vi "Test ZLG_CAN API.vi"() -> ()   [LabVIEW 2020]
doc: "ZLG_CAN API Tester."
uses:
  ZLG_CAN.lvlib
  <userlib>/_OpenG.lib/array/array.llb/Reverse 2D Array (String)__ogtk.vi
  CAN_CYCLE.vi
  Sources/Global_Variable/Global.vi
panel:
  in  "Test":bool
  in  "Recive_Wait":bool
  out "Cycle_VI":refnum<vi>[](array[refnum])
  in  "CAN_CYCLE":T1(array[cluster]) {"周期(ms)" min=1 format="%d ms"; "ID" format="0x%x"}
  in  "CAN_Recive_Data":string[][](table)
  in  "帧格式":enum8{"数据帧", "远程帧"}(ring)
  in  "帧类型":enum8{"标准帧", "扩展帧"}(ring)
  in  "SENT CAN":bool
  in  "CAN_Frame":string
  in  "ID":u32
  in  "SENT CAN CYCLE":bool
  out "CAN Opening？":bool
  in  "波特率":u32(ring)=11 items=["5Kbps", "10Kbps", "20Kbps", "40Kbps", "50Kbps", "80Kbps", "100Kbps", "125Kbps", "200Kbps", "250Kbps", "400Kbps", "500Kbps", "666Kbps", "800Kbps", "1000Kbps"]
  in  "Close_CAN":bool
  in  "Open_CAN":bool
  in  "通道":u32(ring) items=["0", "1"]
  in  "索引":u32(ring) items=["0", "1", "2", "3", "4", "5", "6", "7", "8"]
  in  "设备类型":u32(ring)=27 items=["PCI5121"=1, "PCI9810"=2, "USBCAN1"=3, "USBCAN2"=4, "PCI9820"=5, "PCI5110"=7, "PC104CAN"=11, "CANETUDP"=12, "PCI9840B"=14, "PC104C2"=15, "PCI9820I"=16, "CANETTCP"=17, "PCIE9221"=24, "PCI5010U"=19, "USBCAN_E_U"=20, "USBCAN_2E_U"=21, "PCI5020U"=22, "PCIE9120I"=27, "PCIE9110I"=28, "PCIE9140I"=29]
  in  "Show Block Diagram":bool
  in  "Stop Module":bool
  in  "Start Module":bool
  in  "Hide Module Panel":bool
  in  "Show Module Panel":bool
  out "Status":string
  out "Module Running?":bool
  # "This VI tests the API for the Module."
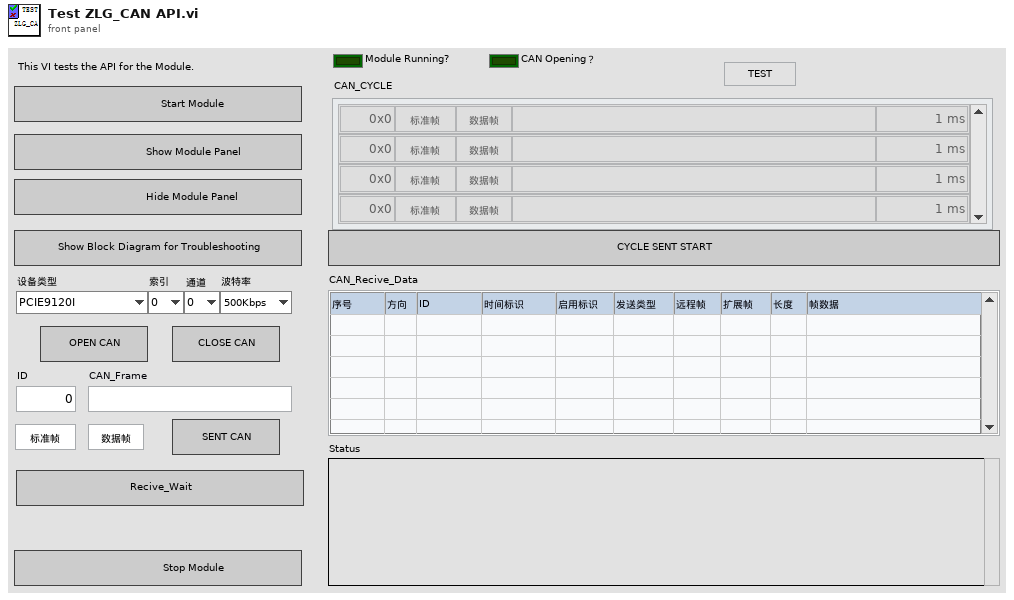
[diagram p1: front panel]
types:
  T1 = cluster{"ID":u32, "帧类型":enum8{"标准帧", "扩展帧"}, "帧格式":enum16{"数据帧", "远程帧"}, "帧数据":string, "周期(ms)":u32}[]
  T2 = typedef "ZLG_CAN.lvlib/Broadcast Events--cluster.ctl" = cluster{"Module Did Init":refnum<user-event>, "Status Updated":refnum<user-event>, "Error Reported":refnum<user-event>, "Module Did Stop":refnum<user-event>, "Update Module Execution Status":refnum<user-event>, "CAN_Recive":refnum<user-event>}
  T3 = enum32{"Invalid", "Standard", "Closed", "Hidden", "Minimized", "Maximized"}
  T4 = typedef "ZLG_CAN.lvlib/Start_CAN (Reply Payload)--cluster.ctl" = cluster{"Success":bool, "Start_CAN_error":errorcluster}
  T5 = typedef "ZLG_CAN.lvlib/CAN_Frame.ctl" = cluster{"[0]":u8, "[1]":u8, "[2]":u8, "[3]":u8, "[4]":u8, "[5]":u8, "[6]":u8, "[7]":u8}
  T6 = typedef "ZLG_CAN.lvlib/CAN_OBJ_R.ctl" = cluster{"ID":u32, "TimeStamp":u32, "TimeFlag":u8, "SendType":u8, "RemoteFlag":u8, "ExternFlag":u8, "DataLen":u8, "数值":u8, "数值":u8, "数值":u8, "数值":u8, "数值":u8, "数值":u8, "数值":u8, "数值":u8, "数值":u8, "数值":u8, "数值":u8}
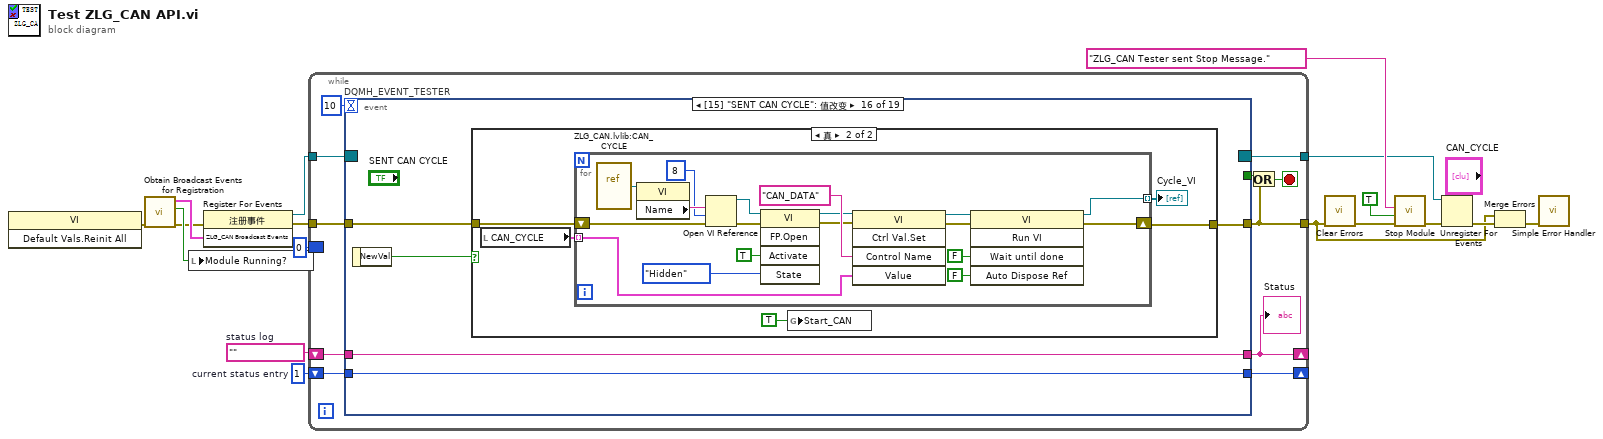
[diagram p0: block diagram]
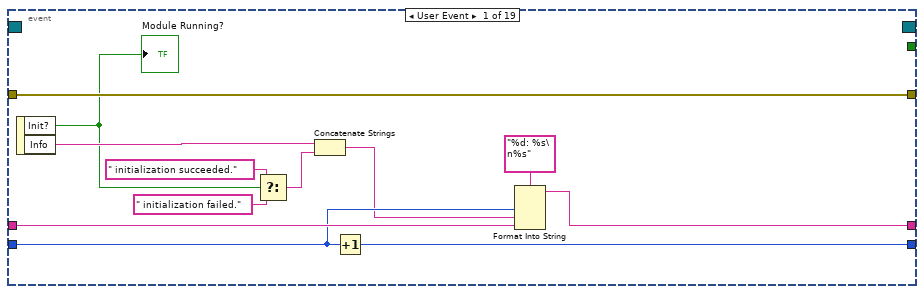
[diagram p2: hidden frame]
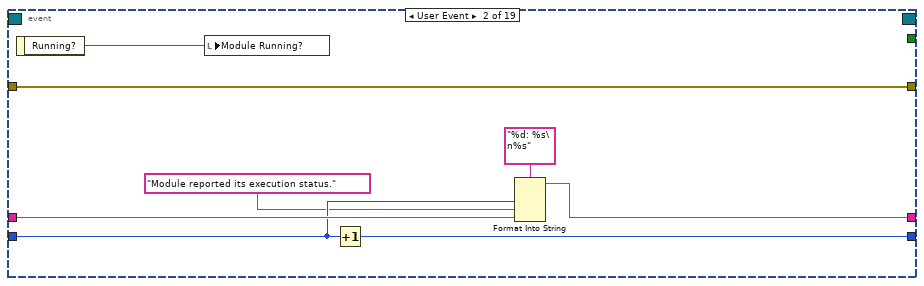
[diagram p3: hidden frame]
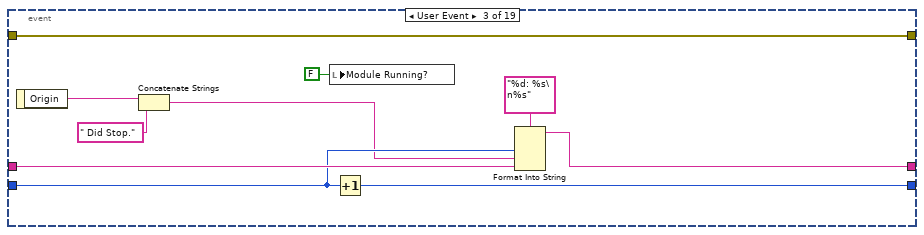
[diagram p4: hidden frame]
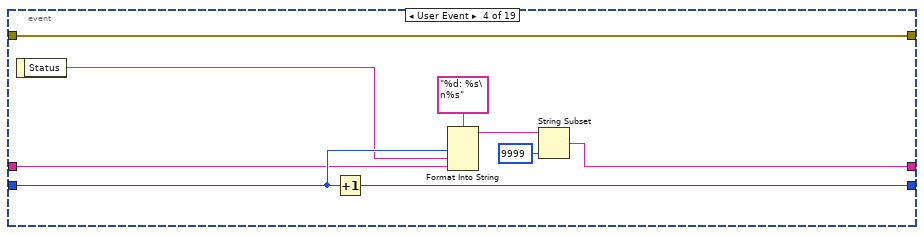
[diagram p5: hidden frame]
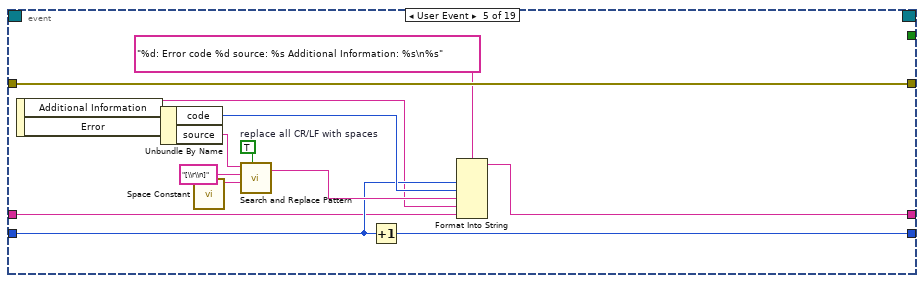
[diagram p6: hidden frame]
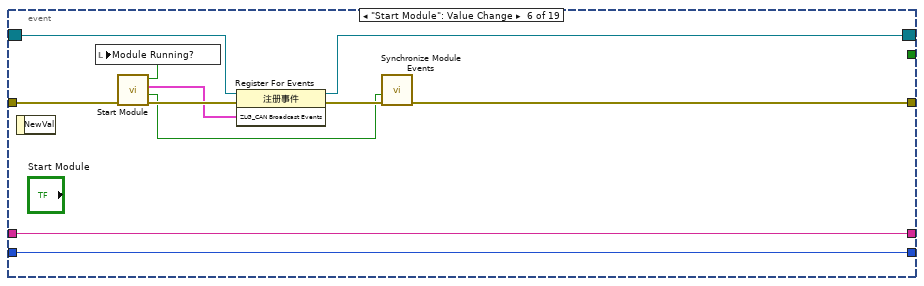
[diagram p7: hidden frame]
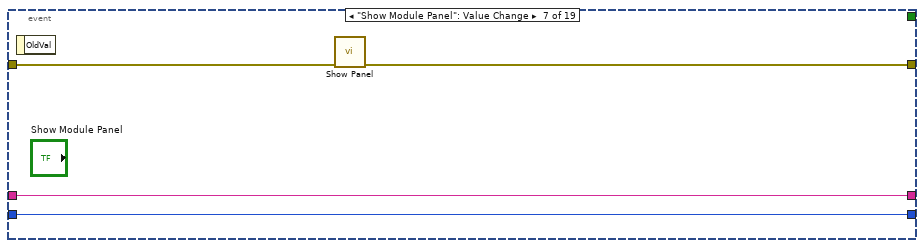
[diagram p8: hidden frame]
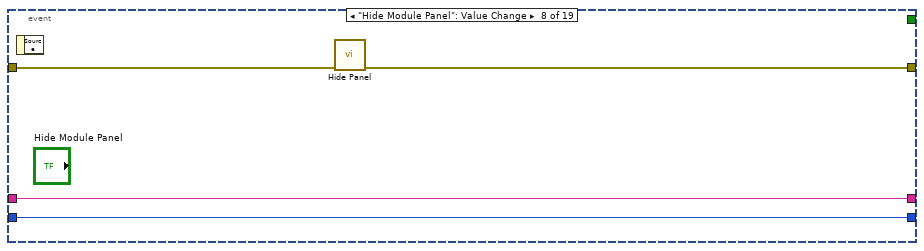
[diagram p9: hidden frame]
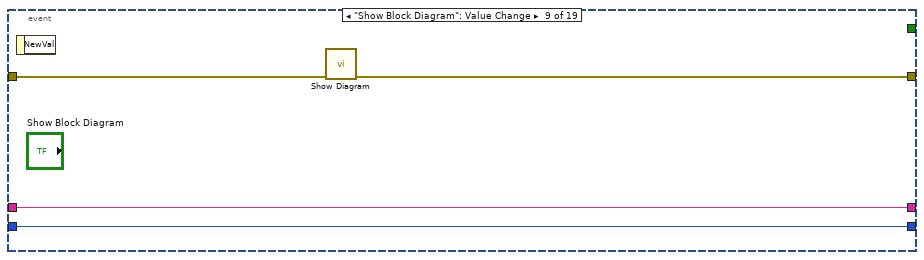
[diagram p10: hidden frame]
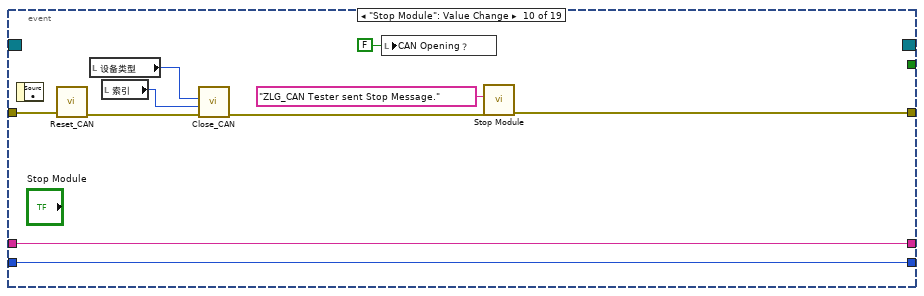
[diagram p11: hidden frame]
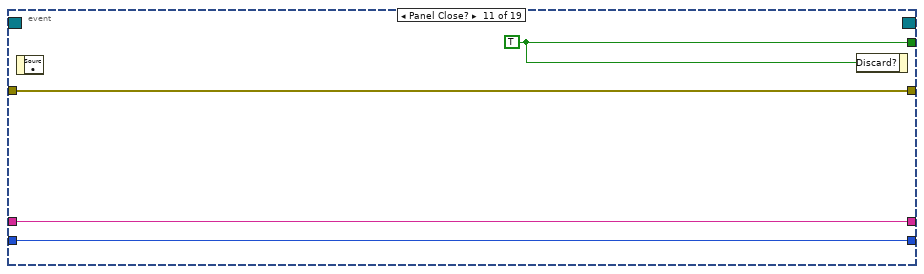
[diagram p12: hidden frame]
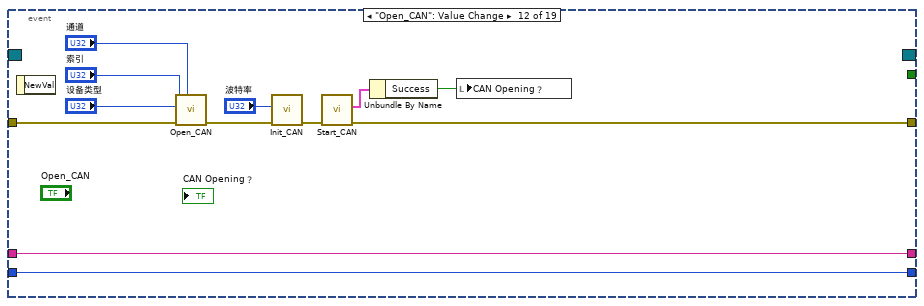
[diagram p13: hidden frame]
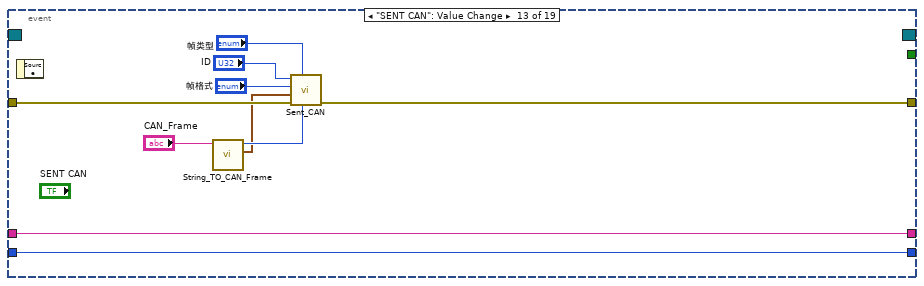
[diagram p14: hidden frame]
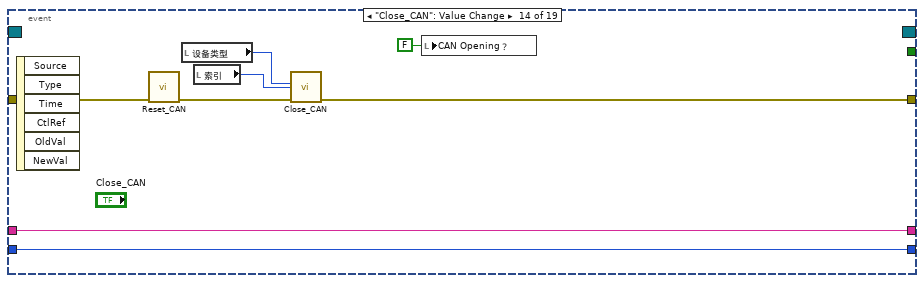
[diagram p15: hidden frame]
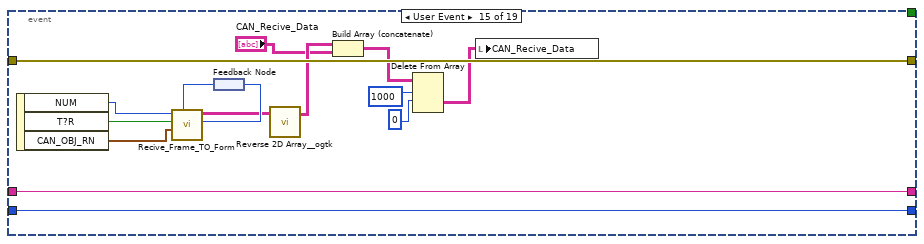
[diagram p16: hidden frame]
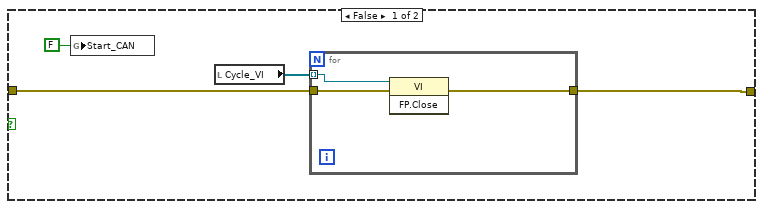
[diagram p17: hidden frame]
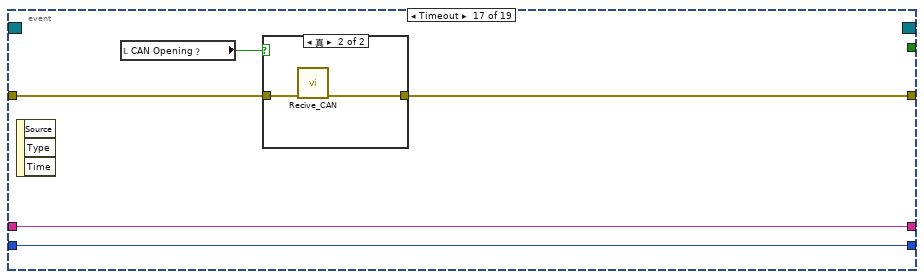
[diagram p18: hidden frame]
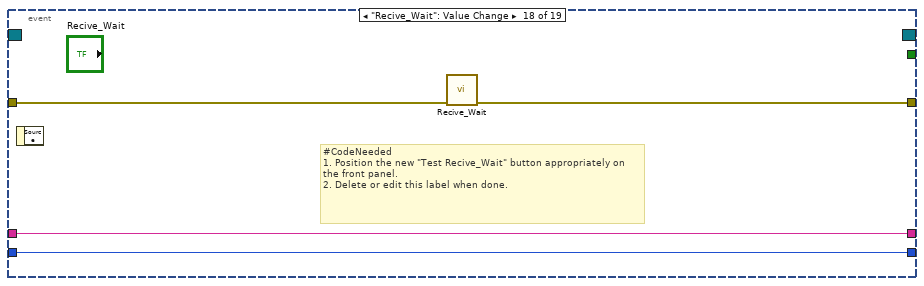
[diagram p20: hidden frame]
diagram:
  w13 = 1  # current status entry
  w14 = ""  # status log
  n1 = invoke class="VI" method="Default Vals.Reinit All"() -> (error out=w3:errorcluster)  [unwired: 3 in, 2 out]
  n2 = call "Obtain Broadcast Events for Registration.vi"("error in (no error)"=w3) -> ("error out"=w2:errorcluster, "Already running?"=w4:bool, "ZLG_CAN Broadcast Events"=w11:T2)  [unwired: 8 in]
  n3 = local write "Module Running?"(w4) -> ()
  n4 = register-events(error in=w2, w11) -> (reference out=w10:refnum<event-registration>, error out=w12:errorcluster)  [unwired: 1 in]
  n5 = while {
    tunnel: w10 -> [w28]
    tunnel: [w20] -> w5
    shift-right: [w19] -> _
    shift-left: w14 -> [w25]
    shift-right: [w24] -> _
    shift-left: w13 -> [w26]
    tunnel: w12 -> [w22]
    tunnel: [w21] -> w9
    border: u32 0 ("TRCount Out") -> [_]
    stop <- w23 stop-if-true
    n6 = event "DQMH_EVENT_TESTER" shown="[15] \"SENT CAN CYCLE\": 值改变" {
      selector: w28 -> [_ _ _ _ _ w86 _ _ _ _ _ _ _ _ _ _ _ _ _]
      dyn-events: [_ _ _ _ _ w85 _ _ _ _ _ _ _ _ _ _ _ _ _] -> w21
      timeout: 10 -> [_ _ _ _ _ _ _ _ _ _ _ _ _ _ _ _ _ _ _]
      tunnel: [_ _ _ _ _ _ _ _ _ _ w118 _ _ _ _ _ _ _ _] -> w27
      tunnel: [w40 w42 w49 w62 w81 w84 w96 w100 w101 w112 w115 w124 w137 w146 w163 w165 w200 w207 w217] -> w20
      tunnel: w26 -> [w37 w46 w56 w65 w71 w89 w94 w98 w102 w113 w116 w129 w138 w147 w161 w167 w201 w208 w215]
      tunnel: w25 -> [w38 w47 w57 w64 w69 w90 w95 w99 w103 w114 w117 w130 w139 w148 w162 w168 w202 w209 w216]
      tunnel: [w35 w44 w54 w61 w72 w90 w95 w99 w103 w114 w117 w130 w139 w148 w162 w168 w202 w209 w216] -> w19
      tunnel: [w36 w45 w55 w67 w70 w89 w94 w98 w102 w113 w116 w129 w138 w147 w161 w167 w201 w208 w215] -> w24
      tunnel: w22 -> [w40 w42 w49 w62 w81 w83 w93 w97 w104 w109 w115 w119 w140 w142 w163 w166 w203 w210 w217]
      event User Event {
        n7 = event-data() -> ("Init?"=w32:bool, "Info"=w34:string)  [unwired: 1 in]
        "Module Running?" <- w32
        n8 = Select(t=" initialization succeeded.", s=w32, f=" initialization failed.") -> (s? t:f=w29:string)
        n9 = Concatenate Strings(w34, w29) -> (w33:string)
        n10 = Increment(x=w37) -> (x+1=w36:i32)
        n11 = Format Into String(format string="%d: %s\n%s", w37, w33, w38) -> (resulting string=w35:string)  [unwired: 2 in, 1 out]
      }
      event User Event {
        n12 = event-data() -> ("Running?"=w41:bool)  [unwired: 1 in]
        n13 = local write "Module Running?"(w41) -> ()
        n14 = Increment(x=w46) -> (x+1=w45:i32)
        n15 = Format Into String(format string="%d: %s\n%s", w46, "Module reported its execution status.", w47) -> (resulting string=w44:string)  [unwired: 2 in, 1 out]
      }
      event User Event {
        n16 = event-data() -> ("Origin"=w53:string)  [unwired: 1 in]
        n17 = Concatenate Strings(w53, " Did Stop.") -> (w52:string)
        n18 = local write "Module Running?"(FALSE ("Module Did Init?")) -> ()
        n19 = Increment(x=w56) -> (x+1=w55:i32)
        n20 = Format Into String(format string="%d: %s\n%s", w56, w52, w57) -> (resulting string=w54:string)  [unwired: 2 in, 1 out]
      }
      event User Event {
        n21 = event-data() -> ("Status"=w63:string)  [unwired: 1 in]
        n22 = Increment(x=w65) -> (x+1=w67:i32)
        n23 = Format Into String(format string="%d: %s\n%s", w65, w63, w64) -> (resulting string=w60:string)  [unwired: 2 in, 1 out]
        n24 = String Subset(string=w60, length (rest)=9999 ("长度（剩余）")) -> (substring=w61:string)  [unwired: 1 in]
      }
      event User Event {
        w77 = TRUE  # replace all CR/LF with spaces
        n25 = event-data() -> ("Additional Information"=w68:string, "Error"=w73:errorcluster)  [unwired: 1 in]
        n26 = Unbundle By Name(w73) -> ("code"=w74:i32, "source"=w75:string)
        n27 = call <vilib>:"Space Constant.vi"() -> ("String"=w78:string)
        n28 = call <vilib>:"Search and Replace Pattern.vi"("string"=w75, "regular expression (\"\")"="[\\r\\n]" ("regular expression (\"\")"), "replace string (\"\")"=w78, "replace all? (F)"=w77) -> ("result string"=w76:string)  [unwired: 1 in, 1 out]
        n29 = Increment(x=w71) -> (x+1=w70:i32)
        n30 = Format Into String(format string="%d: Error code %d source: %s Additional Information: %s\n%s", w71, w74, w76, w68, w69) -> (resulting string=w72:string)  [unwired: 2 in, 1 out]
      }
      event "Start Module": Value Change {
        n31 = event-data() -> ()  [unwired: 1 in, 1 out]
        n32 = call "Start Module.vi"("error in (no error)"=w83) -> ("error out"=w91:errorcluster, "Wait for Event Sync?"=w88:bool, "ZLG_CAN Broadcast Events"=w87:T2, "Module Was Already Running?"=w82:bool)  [unwired: 7 in]
        n33 = local write "Module Running?"(w82) -> ()
        n34 = register-events(reference=w86, error in=w91, w87) -> (reference out=w85:refnum<event-registration>, error out=w92:errorcluster)
        n35 = call "Synchronize Module Events.vi"("error in (no error)"=w92, "Wait for Event Sync?"=w88) -> ("error out"=w84:errorcluster)  [unwired: 9 in]
      }
      event "Show Module Panel": Value Change {
        n36 = event-data() -> ()  [unwired: 1 in, 1 out]
        n37 = call "Show Panel.vi"("error in (no error)"=w93) -> ("error out"=w96:errorcluster)  [unwired: 10 in]
      }
      event "Hide Module Panel": Value Change {
        n38 = event-data() -> ()  [unwired: 1 in, 1 out]
        n39 = call "Hide Panel.vi"("error in (no error)"=w97) -> ("error out"=w100:errorcluster)  [unwired: 10 in]
      }
      event "Show Block Diagram": Value Change {
        n40 = event-data() -> ()  [unwired: 1 in, 1 out]
        n41 = call "Show Diagram.vi"("error in (no error)"=w104) -> ("error out"=w101:errorcluster)  [unwired: 10 in]
      }
      event "Stop Module": Value Change {
        n42 = event-data() -> ()  [unwired: 1 in, 1 out]
        n43 = call "Reset_CAN.vi"("error in (no error)"=w109) -> ("error out"=w108:errorcluster)  [unwired: 10 in]
        n44 = local read "设备类型"() -> (w110:u32)
        n45 = local read "索引"() -> (w106:u32)
        n46 = call "Close_CAN.vi"("error in (no error)"=w108, "索引"=w106, "设备类型"=w110) -> ("error out"=w107:errorcluster)  [unwired: 8 in]
        n47 = local write "CAN Opening？"(FALSE ("CAN Opening？")) -> ()
        n48 = call "Stop Module.vi"("error in (no error)"=w107, "Origin"="ZLG_CAN Tester sent Stop Message.") -> ("error out"=w112:errorcluster)  [unwired: 9 in]
      }
      event Panel Close? {
        w118 = TRUE ("Discard?")
        n49 = event-data() -> ()  [unwired: 1 in, 1 out]
        n50 = event-data("Discard?"=w118) -> ()  [unwired: 1 in, 1 out]
      }
      event "Open_CAN": Value Change {
        n51 = event-data() -> ()  [unwired: 1 in, 1 out]
        n52 = call "Open_CAN.vi"("CAN 通道"="通道", "error in (no error)"=w119, "索引"="索引", "设备类型"="设备类型") -> ("error out"=w127:errorcluster)  [unwired: 7 in]
        n53 = call "Init_CAN.vi"("error in (no error)"=w127, "波特率"="波特率") -> ("error out"=w125:errorcluster)  [unwired: 9 in]
        n54 = call "Start_CAN.vi"("error in (no error)"=w125) -> ("error out"=w124:errorcluster, "Reply Payload"=w121:T4)  [unwired: 8 in, 1 out]
        n55 = Unbundle By Name(w121) -> ("Success"=w120:bool)
        n56 = local write "CAN Opening？"(w120) -> ()
      }
      event "SENT CAN": Value Change {
        n57 = event-data() -> ()  [unwired: 1 in, 1 out]
        n58 = call "String_TO_CAN_Frame.vi"("CAN_Frame"="CAN_Frame") -> ("CAN_FRAME"=w131:T5, "DATA_LEN"=w132:i32)  [unwired: 9 in]
        n59 = call "Sent_CAN.vi"("帧长度"=w132, "帧类型"="帧类型", "error in (no error)"=w140, "帧数据"=w131, "帧格式"="帧格式", "ID"="ID") -> ("error out"=w137:errorcluster)  [unwired: 5 in]
      }
      event "Close_CAN": Value Change {
        n60 = event-data() -> ()  [unwired: 1 in, 6 out]
        n61 = call "Reset_CAN.vi"("error in (no error)"=w142) -> ("error out"=w141:errorcluster)  [unwired: 10 in]
        n62 = local read "设备类型"() -> (w145:u32)
        n63 = local read "索引"() -> (w144:u32)
        n64 = call "Close_CAN.vi"("error in (no error)"=w141, "索引"=w144, "设备类型"=w145) -> ("error out"=w146:errorcluster)  [unwired: 8 in]
        n65 = local write "CAN Opening？"(FALSE ("CAN Opening？")) -> ()
      }
      event User Event {
        n66 = event-data() -> ("NUM"=w159:u16, "T?R"=w160:bool, "CAN_OBJ_RN"=w158:T6[])  [unwired: 1 in]
        n67 = feedback #1() -> (w156:u32)
        n68 = call "Recive_Frame_TO_Form.vi"("TRCount"=w156, "CAN_OBJ_RN"=w158, "T/R"=w160, "NUM"=w159) -> ("TRCount Out"=w157:u32, "数组"=w155:string[][])  [unwired: 6 in]
        n69 = feedback-in #1(w157) -> ()
        n70 = call-poly <userlib>:"Reverse 2D Array__ogtk.vi"("Array"=w155) -> ("Reversed Array"=w154:string[][])  [unwired: 2 in]
        n71 = Build Array (concatenate)(w154, "CAN_Recive_Data") -> (w152:string[][])
        n72 = Delete From Array(array=w152, length=1000 ("长度"), index (row)=0 ("索引 (行)")) -> (deleted portion=w149:string[][])  [unwired: 1 in, 1 out]
        n73 = local write "CAN_Recive_Data"(w149) -> ()
      }
      event "SENT CAN CYCLE": Value Change {
        n74 = event-data() -> ("NewVal"=w164:bool)  [unwired: 1 in]
        n75 = case shown="真" w164 {
          tunnel: w166 -> [w170 w179]
          tunnel: [w169 w178] -> w165
          frame False {
            n76 = global write "Global.vi" "Start_CAN"(FALSE ("STOP_CAN")) -> ()
            n77 = local read "Cycle_VI"() -> (w171:refnum<vi>[])
            n78 = for {
              tunnel: w171 -> [w175] mode=indexing
              tunnel: w170 -> [w174]
              tunnel: [w173] -> w169
              n79 = invoke class="VI" method="FP.Close"(reference=w175, error in=w174) -> (error out=w173:errorcluster)  [unwired: 1 in, 2 out]
            }
          }
          frame True {
            n80 = local read "CAN_CYCLE"() -> (w180:T1)
            n81 = for {
              tunnel: w180 -> [w192] mode=indexing
              shift-right: [w184] -> w178
              shift-left: w179 -> [w195]
              tunnel: [w183] -> w177 mode=indexing
              n82 = vi-ref "ZLG_CAN.lvlib:CAN_CYCLE.vi"() -> (w198:refnum<vi>)
              n83 = property class="VI"(reference=w198) -> ("Name"=w197:string)  [unwired: 1 in, 2 out]
              n84 = Open VI Reference(vi path=w197, options=8 ("选项"), error in (no error)=w195) -> (vi reference=w194:refnum<vi>, error out=w190:errorcluster)  [unwired: 3 in]
              n85 = invoke class="VI" method="FP.Open"(reference=w194, error in=w190, "Activate"=TRUE ("激活？"), "State"=T3."Hidden" ("状态")) -> (reference out=w191:refnum<vi>, error out=w189:errorcluster)  [unwired: 1 in, 3 out]
              n86 = invoke class="VI" method="Ctrl Val.Set"(reference=w191, error in=w189, "Control Name"="CAN_DATA" ("控件名"), "Value"=w192) -> (reference out=w186:refnum<vi>, error out=w185:errorcluster)  [unwired: 1 in, 3 out]
              n87 = invoke class="VI" method="Run VI"(reference=w186, error in=w185, "Wait until done"=FALSE ("结束前等待"), "Auto Dispose Ref"=FALSE ("自动销毁引用")) -> (reference out=w183:refnum<vi>, error out=w184:errorcluster)  [unwired: 1 in, 3 out]
            }
            "Cycle_VI" <- w177
            n88 = global write "Global.vi" "Start_CAN"(TRUE ("STOP_CAN")) -> ()
          }
        }
      }
      event Timeout {
        n89 = event-data() -> ()  [unwired: 1 in, 3 out]
        n90 = local read "CAN Opening？"() -> (w199:bool)
        n91 = case shown="真" w199 {
          tunnel: w203 -> [w204 w206]
          tunnel: [w204 w205] -> w200
          frame False {
          }
          frame True {
            n92 = call "Recive_CAN.vi"("error in (no error)"=w206) -> ("error out"=w205:errorcluster)  [unwired: 10 in]
          }
        }
      }
      event "Recive_Wait": Value Change {
        # "#CodeNeeded\n1. Position the new \"Test Recive_Wait\" button appropriately on the front panel.\n2. Delete or edit this label when done."
        n93 = event-data() -> ()  [unwired: 1 in, 1 out]
        n94 = call "Recive_Wait.vi"("error in (no error)"=w210) -> ("error out"=w207:errorcluster)  [unwired: 8 in, 2 out]
      }
      event "Test": Value Change {
        n95 = event-data() -> ()  [unwired: 1 in, 6 out]
        n96 = vi-ref "读取版本号.vi"() -> (w214:refnum<vi>)
        n97 = call "CallVI.vi"("VI引用"=w214, "状态"=T3."Standard") -> ("VI引用OUT"=w211:refnum<vi>)  [unwired: 12 in, 1 out]
        n98 = property class="VI"(reference=w211, "BDWin.Open"=TRUE ("程序框图窗口:打开")) -> ()  [unwired: 1 in, 2 out]
      }
    }
    "Status" <- w19
    n99 = Or(x=w27, y=w20) -> (x .or. y?=w23:bool)
  }
  n100 = call <vilib>:"Clear Errors.vi"("error in (no error)"=w5) -> ("error out"=w7:errorcluster)  [unwired: 5 in, 1 out]
  n101 = call "Stop Module.vi"("error in (no error)"=w7, "Wait for Module to Stop? (F)"=TRUE ("Wait for Module to stop?"), "Origin"="ZLG_CAN Tester sent Stop Message.") -> ("error out"=w16:errorcluster)  [unwired: 8 in]
  n102 = Unregister For Events(event registration refnum=w9, error in=w16) -> (error out=w17:errorcluster)
  n103 = Merge Errors(w5, w17) -> (w6:errorcluster)
  n104 = call <vilib>:"Simple Error Handler.vi"("error in (no error)"=w6) -> ()  [unwired: 4 in, 5 out]
